vi "VNA - Initiate and Fetch Single Site.vi"(8 "error in (no error)":errorcluster, 10 "Pins":string[](array[string])=["RF1", "RF2"], 11 "Semiconductor Module Context":T1) -> (0 "error out":errorcluster, 1 "P2_Capacitance":dbl[](array[numeric]), 2 "P1_Capacitance":dbl[](array[numeric]), 3 "Semiconductor Module Context Out":T1, 4 "S22":string[](array[string]), 6 "S11":string[](array[string]))   [LabVIEW 2013]
doc: "Initiates and fetches niVNA S11 measurements and converts it to a capacitance measurement."
uses:
  <vilib>/NI_TestStand_SemiconductorModule/NI_TestStand_Semiconductor_Module.lvlibp/PinMap/General/SemiconductorModuleContext.ctl
  <vilib>/Analysis/baseanly.llb/Mean (DBL).vi
  <instrlib>/niVNA/niVNA.llb/niVNA Fetch Sweep Measurement Complex (CDB).vi
  <vilib>/Analysis/baseanly.llb/Mean (CDB).vi
  Pin Map API/VNA Custom Instrument.lvlib
  <vilib>/Analysis/NI_AALBase.lvlib
  <vilib>/NI_TestStand_SemiconductorModule/NI_TestStand_Semiconductor_Module.lvlibp
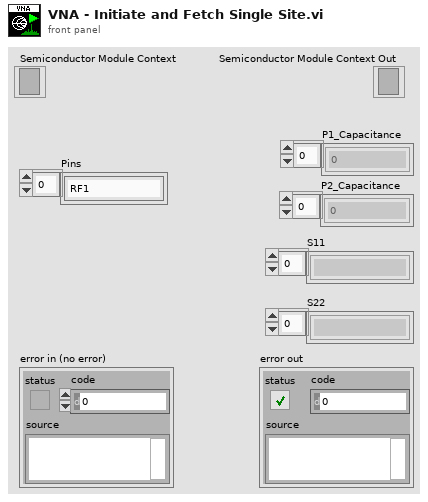
[diagram p1: front panel]
types:
  T1 = typedef "NI_TestStand_Semiconductor_Module.lvlibp/SemiconductorModuleContext.ctl" = refnum<k7>
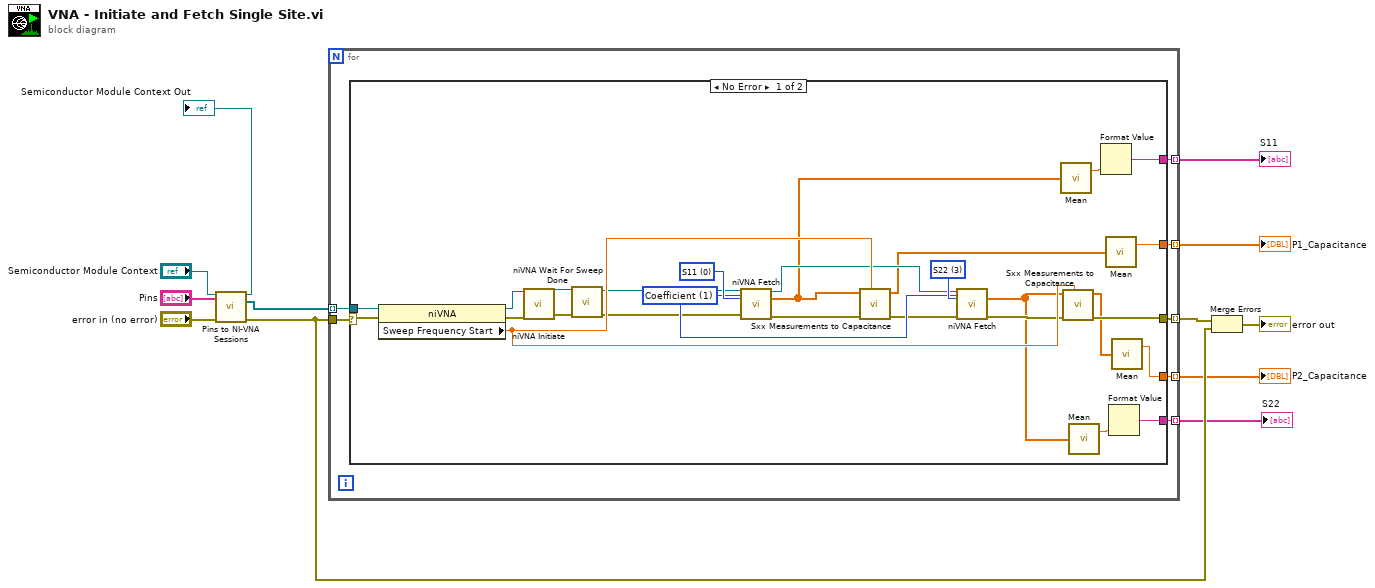
[diagram p0: block diagram]
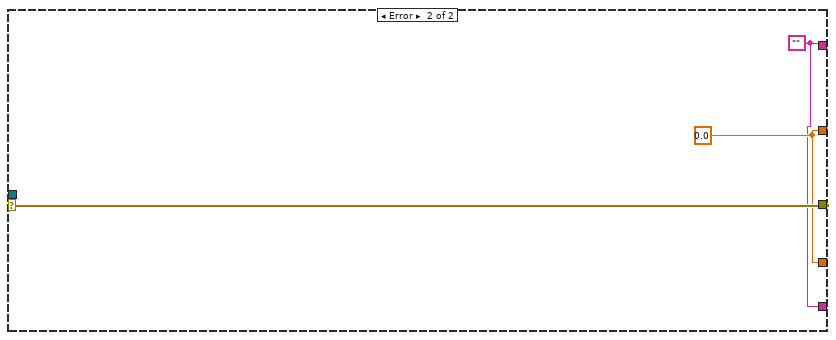
[diagram p2: hidden frame]
diagram:
  n1 = call "Pins to NI-VNA Sessions.vi"("Semiconductor Module Context"="Semiconductor Module Context", "Pins"="Pins", "error in (no error)"="error in (no error)") -> ("Semiconductor Module Context Out"=→"Semiconductor Module Context Out":T1, "Instrument Sessions"=w3:refnum<k15>[], "error out"=w8:errorcluster)  [unwired: 8 in, 2 out]
  n2 = for {
    tunnel: [w19] -> w9 mode=indexing
    tunnel: w8 -> [w18]
    tunnel: [w17] -> w5 mode=indexing
    tunnel: [w16] -> w4 mode=indexing
    tunnel: w3 -> [w15] mode=indexing
    tunnel: [w14] -> w2 mode=indexing
    tunnel: [w13] -> w1 mode=indexing
    n3 = case shown="No Error" w18 {
      selector: w18 -> [w46 w49]
      tunnel: [w35 w49] -> w19
      tunnel: [w27 w48] -> w17
      tunnel: [w28 w48] -> w16
      tunnel: w15 -> [w26 _]
      tunnel: [w23 w47] -> w14
      tunnel: [w20 w47] -> w13
      frame No Error {
        w40 = 1 items=["Impedance", "Coefficient"] ("format")
        w41 = 0 items=["S11", "S21", "S12", "S22"] ("measurement")
        w42 = 3 items=["S11", "S21", "S12", "S22"] ("measurement")
        n4 = property class="niVNA"(reference=w26, error in=w46) -> (reference out=w45:refnum<k15>, error out=w44:errorcluster, "Sweep Frequency Start"=w43:dbl)
        n5 = call <instrlib>:"niVNA Initiate.vi"("instrument handle"=w45, "error in"=w44) -> ("instrument handle out"=w34:refnum<k15>, "error out"=w33:errorcluster)  [unwired: 12 in]
        n6 = call <instrlib>:"niVNA Wait For Sweep Done.vi"("instrument handle"=w34, "error in"=w33) -> ("instrument handle out"=w31:refnum<k15>, "error out"=w32:errorcluster)  [unwired: 12 in]
        n7 = call-poly <instrlib>:"niVNA Fetch.vi"("instrument handle"=w31, "measurement"=w41, "format"=w40, "error in"=w32) -> ("instrument handle out"=w38:refnum<k15>, "data"=w25:cdb[], "error out"=w37:errorcluster)  [unwired: 8 in, 1 out]
        n8 = call "Sxx Measurements to Capacitance.vi"("Sweep Frequency Start"=w43, "error in (no error)"=w37, "S11 Data"=w25) -> ("error out"=w36:errorcluster, "Capacitance"=w30:dbl[])  [unwired: 7 in]
        n9 = call-poly <instrlib>:"niVNA Fetch.vi"("instrument handle"=w38, "measurement"=w42, "format"=w40, "error in"=w36) -> ("data"=w21:cdb[], "error out"=w39:errorcluster)  [unwired: 8 in, 2 out]
        n10 = call-poly <vilib>:"Mean.vi"("X"=w25) -> ("mean"=w24:cdb)  [unwired: 1 out]
        n11 = call "Sxx Measurements to Capacitance.vi"("Sweep Frequency Start"=w43, "error in (no error)"=w39, "S11 Data"=w21) -> ("error out"=w35:errorcluster, "Capacitance"=w29:dbl[])  [unwired: 7 in]
        n12 = call-poly <vilib>:"Mean.vi"("X"=w21) -> ("mean"=w22:cdb)  [unwired: 1 out]
        n13 = Format Value(value (0)=w24) -> (output string=w23:string)  [unwired: 2 in]
        n14 = call-poly <vilib>:"Mean.vi"("X"=w30) -> ("mean"=w27:dbl)  [unwired: 1 out]
        n15 = Format Value(value (0)=w22) -> (output string=w20:string)  [unwired: 2 in]
        n16 = call-poly <vilib>:"Mean.vi"("X"=w29) -> ("mean"=w28:dbl)  [unwired: 1 out]
      }
      frame Error {
        w47 = ""
        w48 = 0.0
      }
    }
  }
  "P1_Capacitance" <- w5
  "P2_Capacitance" <- w4
  "S11" <- w2
  "S22" <- w1
  n17 = Merge Errors(w9, w8) -> (→"error out":errorcluster)
